vi "Configure Waveform (Trapezoid).vi"(0 "VISA resource name":refnum<visa-resource-name>, 1 "Start Level (0)":dbl, 2 "Start Time (0 second)":dbl, 3 "Rise Time (0 second)":dbl, 5 "Output Channel (0: Channel 1)":i32(ring) items=["Channel 1", "Channel 2"], 7 "Source Mode (1: Voltage)":i32(ring)=1 items=["Current", "Voltage"], 9 "Top Time (0 second)":dbl, 11 "error in (no error)":errorcluster, 12 "Top Level (0)":dbl, 13 "End Time (0 second)":dbl, 14 "Fall Time (0 second)":dbl) -> (4 "VISA resource name out":refnum<visa-resource-name>, 15 "error out":errorcluster)   [LabVIEW 2026, in "Agilent B2900 Series.lvlib"]
doc: "Configure current or voltage trapezoid waveform output.\n\n<B>Note:</B>\nThis VI is only supported by Agilent models B2961A, B2962A, B2961B,B2962B,B2961C and B2962C."
uses:
  Agilent B2900 Series.lvlib
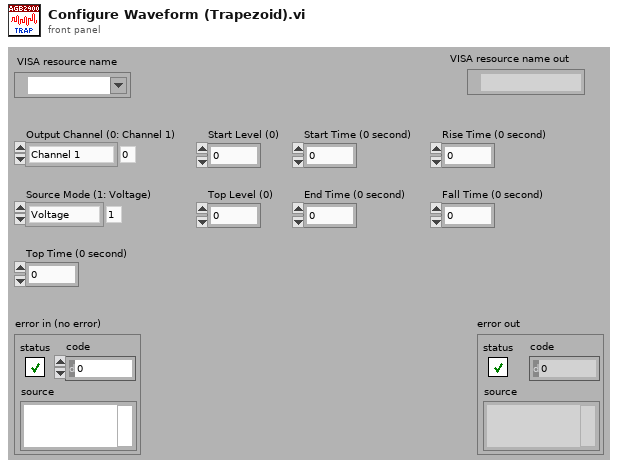
[diagram p1: front panel]
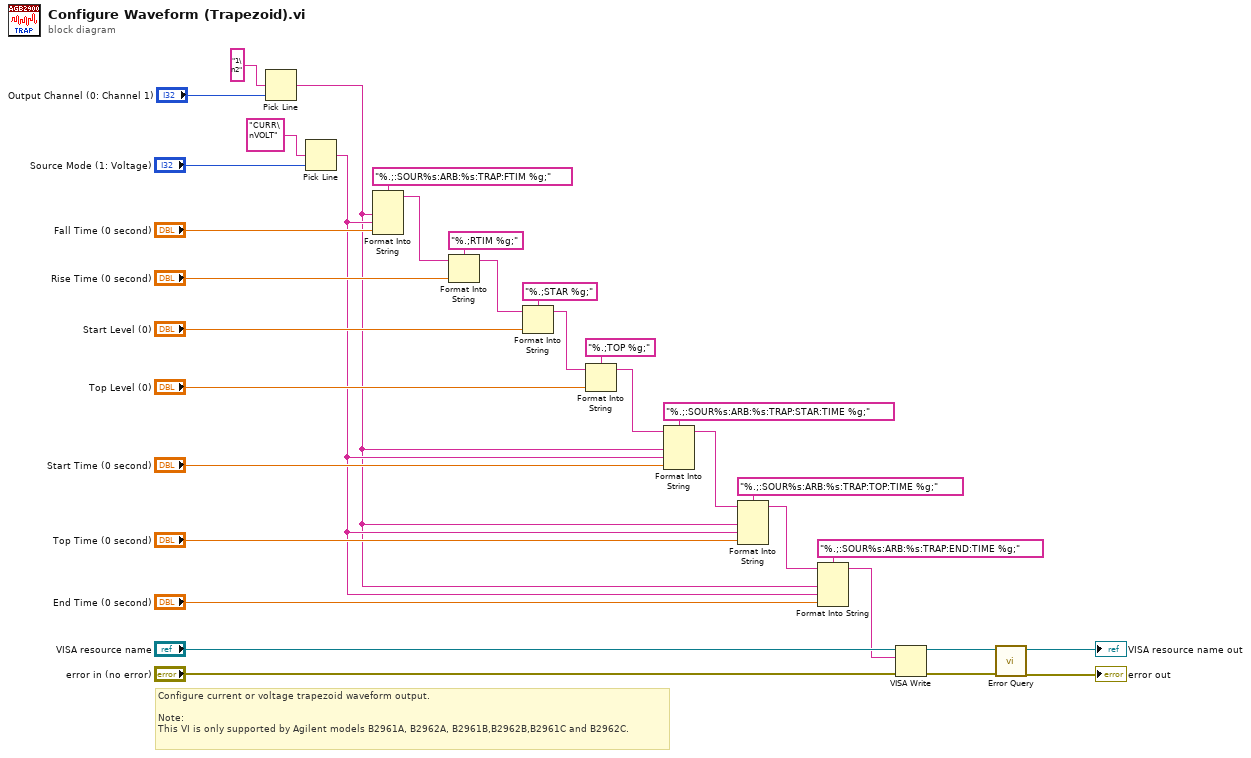
[diagram p0: block diagram]
diagram:
  # "Configure current or voltage trapezoid waveform output.\n\nNote:\nThis VI is only supported by Agilent models B2961A, B2962A, B2961B,B2962B,B2961C and B2962C."
  n1 = Pick Line(multi-line string="1\n2" ("string (\"\")"), line index="Output Channel (0: Channel 1)") -> (output string=w5:string)  [unwired: 1 in]
  n2 = Pick Line(multi-line string="CURR\nVOLT" ("string (\"\")"), line index="Source Mode (1: Voltage)") -> (output string=w6:string)  [unwired: 1 in]
  n3 = Format Into String(format string="%.;:SOUR%s:ARB:%s:TRAP:FTIM %g;", w5, w6, "Fall Time (0 second)") -> (resulting string=w12:string)  [unwired: 2 in, 1 out]
  n4 = Format Into String(format string="%.;RTIM %g;", initial string=w12, "Rise Time (0 second)") -> (resulting string=w11:string)  [unwired: 1 in, 1 out]
  n5 = Format Into String(format string="%.;STAR %g;", initial string=w11, "Start Level (0)") -> (resulting string=w10:string)  [unwired: 1 in, 1 out]
  n6 = Format Into String(format string="%.;TOP %g;", initial string=w10, "Top Level (0)") -> (resulting string=w4:string)  [unwired: 1 in, 1 out]
  n7 = Format Into String(format string="%.;:SOUR%s:ARB:%s:TRAP:STAR:TIME %g;", initial string=w4, w5, w6, "Start Time (0 second)") -> (resulting string=w3:string)  [unwired: 1 in, 1 out]
  n8 = Format Into String(format string="%.;:SOUR%s:ARB:%s:TRAP:TOP:TIME %g;", initial string=w3, w5, w6, "Top Time (0 second)") -> (resulting string=w2:string)  [unwired: 1 in, 1 out]
  n9 = Format Into String(format string="%.;:SOUR%s:ARB:%s:TRAP:END:TIME %g;", initial string=w2, w5, w6, "End Time (0 second)") -> (resulting string=w1:string)  [unwired: 1 in, 1 out]
  n10 = VISA Write(VISA resource name="VISA resource name", write buffer=w1, error in (no error)="error in (no error)") -> (VISA resource name out=w21:refnum<visa-resource-name>, error out=w20:errorcluster)  [unwired: 1 out]
  n11 = call "Error Query.vi"("error in (no error)"=w20, "VISA resource name"=w21) -> ("error out"=→"error out":errorcluster, "VISA resource name out"=→"VISA resource name out":refnum<visa-resource-name>)  [unwired: 8 out]
